vi "read_filter_spec.vi"(11 "File path":path) -> (2 "IIR Filter Cluster":T1 {"Forward Coefficients" format="%#_4g"; "Reverse Coefficients" format="%#_4g"})   [LabVIEW 2010]
uses:
  <vilib>/Utility/file.llb/Read From Spreadsheet File (DBL).vi
panel:
  out "Parsed input":dbl[][](array[numeric]) format="%0.3f"
  # "Read in a filter defined in Matlab with e.g. zkp2sos.  Write it out using:\ndlmwrite('file.dat', sos_matrix, '\\t');\n\nNote that in Labview terminology, with the transfer function b/a, b (the numerator) is  the \"Forward Coefficients\" and a (the denominator) is the \"Reverse Coefficients\"."
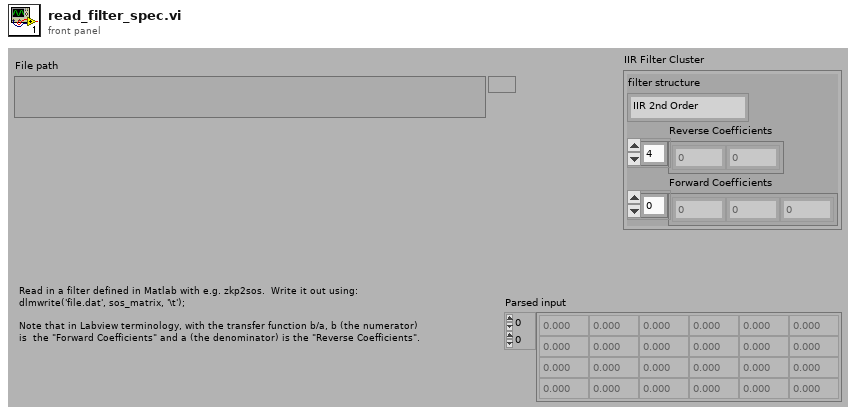
[diagram p1: front panel]
types:
  T1 = cluster{"filter structure":enum32{"IIR 2nd Order", "IIR 4th Order"}, "Reverse Coefficients":dbl[], "Forward Coefficients":dbl[]}
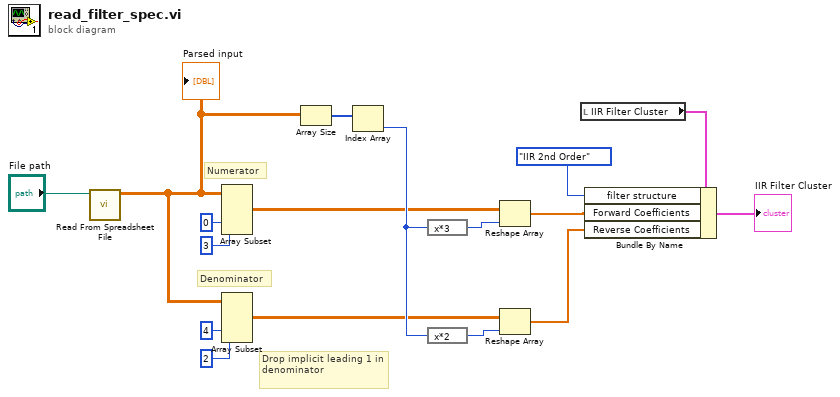
[diagram p0: block diagram]
diagram:
  # "Drop implicit leading 1 in denominator"
  # "Numerator"
  # "Denominator"
  n1 = call-poly <vilib>:"Read From Spreadsheet File.vi"("file path (dialog if empty)"="File path") -> ("all rows"=w7:dbl[][])  [unwired: 3 in, 7 out]
  "Parsed input" <- w7
  n2 = Array Subset(array=w7, index (col)=0 ("length"), length (col)=3 ("length")) -> (w4:dbl[][])  [unwired: 2 in]
  n3 = Array Subset(array=w7, index (col)=4 ("index"), length (col)=2 ("length")) -> (w1:dbl[][])  [unwired: 2 in]
  n4 = Array Size(array=w7) -> (size(s)=w6:i32[])
  n5 = Index Array(array=w6) -> (element=w5:i32)  [unwired: 1 in]
  n6 = expression code="x*3"(w5) -> (w15:i32)
  n7 = expression code="x*2"(w5) -> (w14:i32)
  n8 = Reshape Array(w4, w15) -> (w13:dbl[])
  n9 = Reshape Array(w1, w14) -> (w12:dbl[])
  n10 = local read "IIR Filter Cluster"() -> (w9:T1)
  n11 = Bundle By Name(cluster=w9, "filter structure"=enum32{"IIR 2nd Order", "IIR 4th Order"}."IIR 2nd Order", "Forward Coefficients"=w13, "Reverse Coefficients"=w12) -> (→"IIR Filter Cluster":T1)
